vi "InitDone.vi"(8 "error in (no error)":errorcluster, 10 "Variant":variant, 11 "SLM_Controller in":refnum<class "SLM_Controller.lvclass">) -> (0 "error out":errorcluster, 3 "SLM_Controller out":refnum<class "SLM_Controller.lvclass">)   [LabVIEW 2023, in "SLM_Controller.lvlib" / "SLM_Controller.lvclass"]
uses:
  SLM_Controller.lvclass
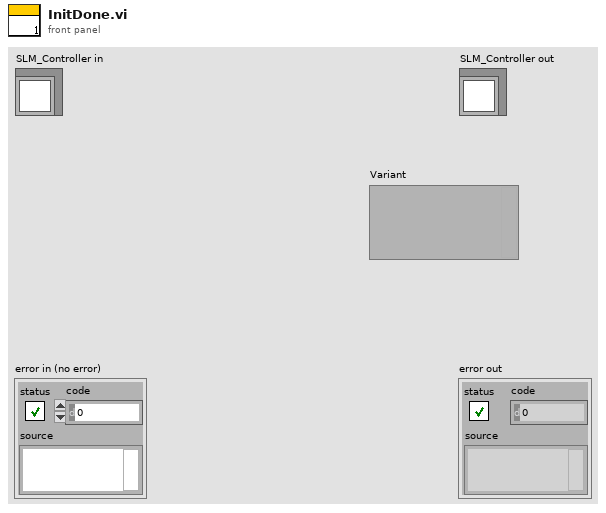
[diagram p1: front panel]
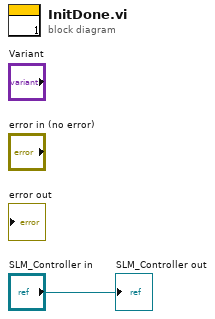
[diagram p0: block diagram]
diagram:
  "SLM_Controller out" <- "SLM_Controller in"
